vi "MECANISMO BOMBA DE AGUA.vi"() -> ()   [LabVIEW 2021]
uses:
  <vilib>/Instr/_visa.llb/VISA Configure Serial Port (Instr).vi
  <vilib>/MakerHub/LINX/Public/Utilities/Open Serial.vi
  <vilib>/LabVIEW Interface for Arduino/LabVIEW Interface for Arduino.lvlib
  <vilib>/MakerHub/LINX/LMH-LINX.lvlib
  <vilib>/MakerHub/LINX/Public/Sensors/Distance/Ultrasonic/Ultrasonic.lvlib
panel:
  out "HUMEDAD 2":dbl
  in  "VISA resource name":refnum<visa-resource-name>
  out "TEMPERATURA":dbl
  out "HUMEDAD":dbl(knob) scale=0.0..255.0
  out "Centimeters":dbl
  out "Slide":dbl(slide) scale=0.0..500.0
  out "BOMBA (6)":bool
  in  "Boolean 4":bool
  out "VALVULA (8)":bool
  in  "Boolean":bool
  out "VALVULA (7)":bool
  in  "stop":bool
  in  "VISA resource":refnum<visa-resource-name>
  # "VÁLVULA 1"
  # "BOMBA DE AGUA"
  # "VÁLVULA 2"
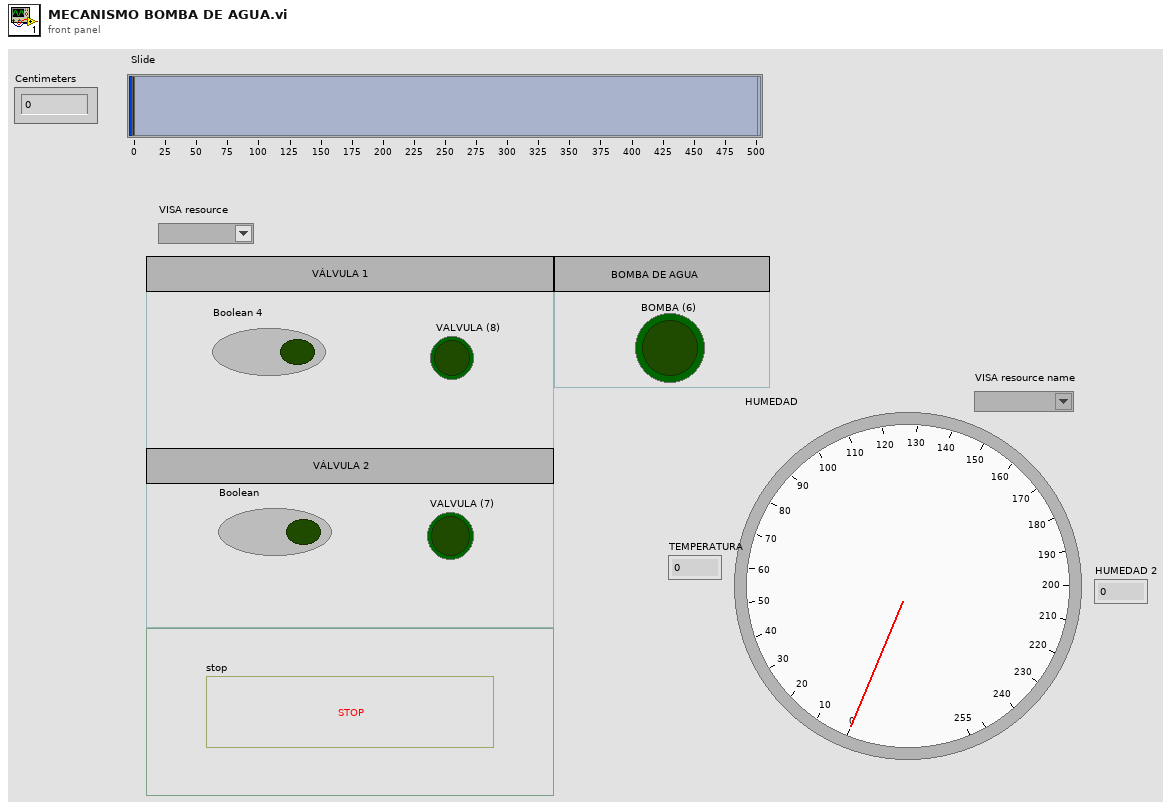
[diagram p1: front panel]
types:
  T1 = typedef "LabVIEW Interface for Arduino.lvlib/Arduino Resource.ctl" = cluster{"VISA resource":refnum<visa-resource-name>, "Board Type":T2, "Connection Type":enum8{"USB / Serial"}, "Bytes Per Packet (15)":u8}
  T2 = typedef "LabVIEW Interface for Arduino.lvlib/Board Type.ctl" = enum16{"Uno", "Dimuelanove w/Atmega 328", "Mega 2560"}
  T3 = typedef "LMH-LINX.lvlib/LINX Ref.ctl" = cluster{"IO":T4, "Interface":T5, "LINX Device Config":T6}
  T4 = typedef "LMH-LINX.lvlib/Platform.ctl" = enum16{"Remote", "Local"}
  T5 = typedef "LMH-LINX.lvlib/Interface.ctl" = enum16{"Serial", "TCP"}
  T6 = typedef "LMH-LINX.lvlib/Device.lvlib/LINX Device Config.ctl" = cluster{"Interface":T5, "COM Port":refnum<visa-resource-name>, "TCP Configuration":T7, "Device Family":u8, "Device ID":u8, "Device Name":string, "TCP Ref":refnum<k5>, "Channels":T8}
  T7 = typedef "LMH-LINX.lvlib/Device.lvlib/TCP Config.ctl" = cluster{"IP Address":string, "Port":u16}
  T8 = typedef "LMH-LINX.lvlib/Channels.ctl" = cluster{"DI":u8[], "DO":u8[], "AI":u8[], "AO":u8[], "PWM":u8[], "QE":u8[], "UART":u8[], "I2C 2":u8[], "SPI":u8[], "CAN":u8[], "Servo":u8[], "AI Ref (V)":dbl, "AI Resolution (Bits)":u8, "AO Ref (V)":dbl, "AO Resolution (Bits)":u8}
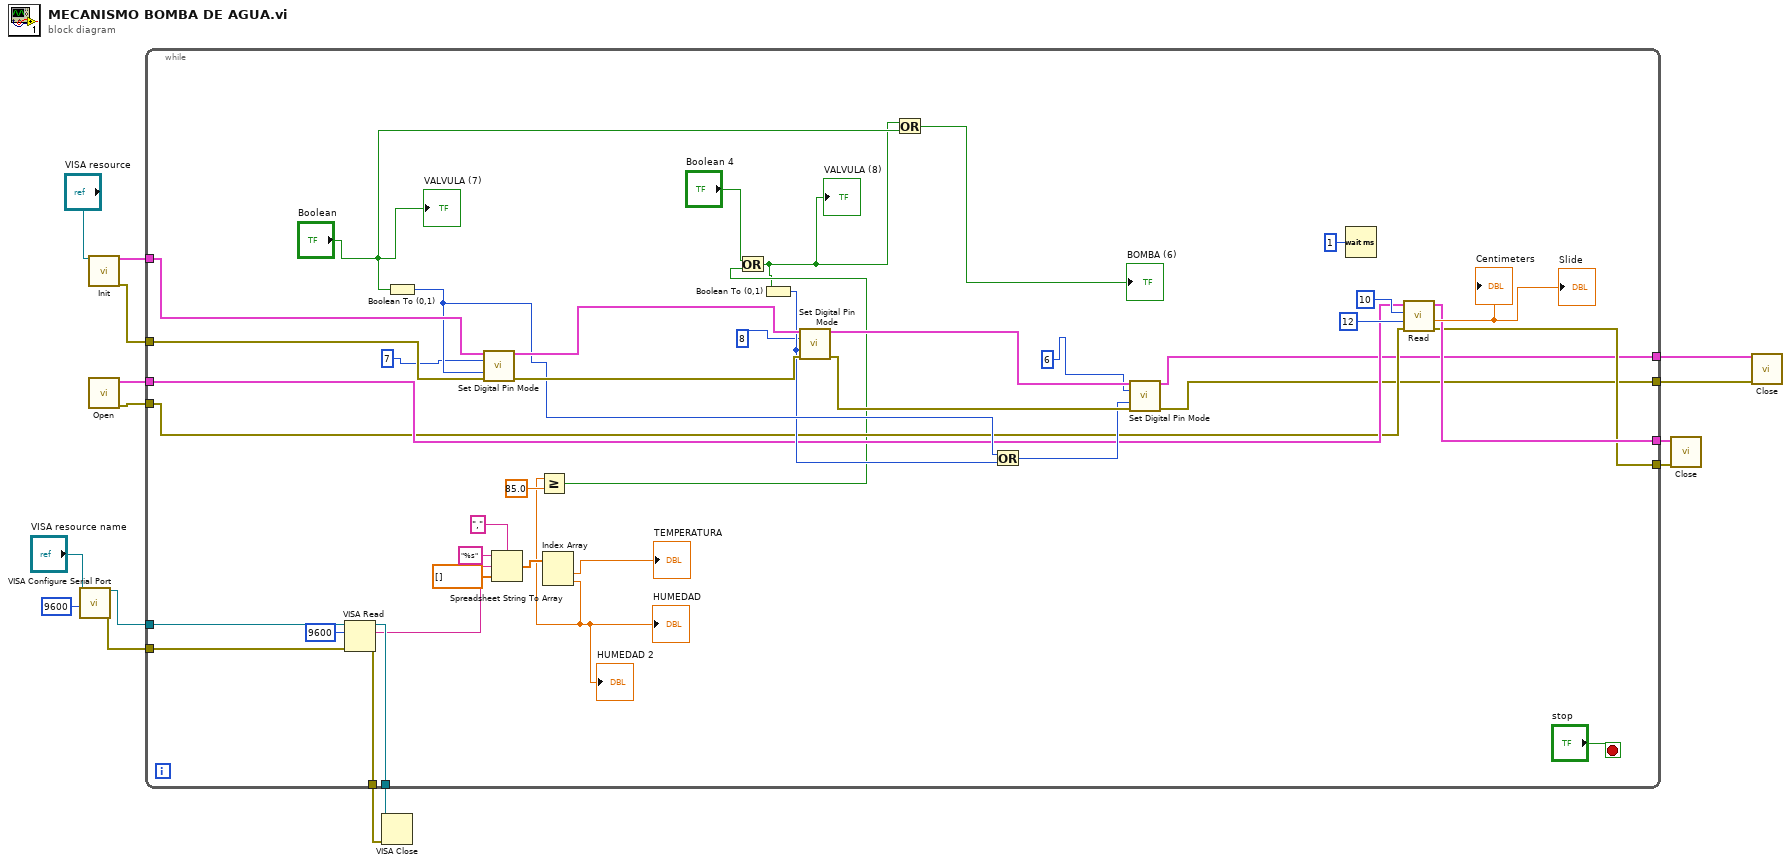
[diagram p0: block diagram]
diagram:
  n1 = call-poly "VISA Configure Serial Port"("VISA resource name"="VISA resource name", "baud rate (9600)"=u32 9600) -> ("VISA resource name out"=w6:refnum<visa-resource-name>, "error out"=w3:errorcluster)  [unwired: 12 in]
  n2 = call <vilib>:"Init.vi"("VISA resource"="VISA resource") -> ("Arduino Resource"=w14:T1, "error out"=w13:errorcluster)  [unwired: 17 in]
  n3 = call-poly <vilib>:"Open.vi"() -> ("Error Out"=w12:errorcluster, "LINX Resource"=w11:T3)  [unwired: 9 in, 1 out]
  n4 = while {
    tunnel: w14 -> [w55]
    tunnel: w13 -> [w54]
    tunnel: w12 -> [w40]
    tunnel: w11 -> [w41]
    tunnel: [w39] -> w10
    tunnel: [w38] -> w9
    tunnel: [w37] -> w8
    tunnel: [w36] -> w7
    tunnel: w6 -> [w35]
    tunnel: [w34] -> w5
    tunnel: [w33] -> w4
    tunnel: w3 -> [w32]
    stop <- "stop" stop-if-true
    n5 = VISA Read(VISA resource name=w35, byte count=u32 9600, error in (no error)=w32) -> (VISA resource name out=w33:refnum<visa-resource-name>, read buffer=w31:string, error out=w34:errorcluster)  [unwired: 1 out]
    n6 = Boolean To (0,1)(Boolean="Boolean") -> (0, 1=w49:i16)
    n7 = call <vilib>:"Set Digital Pin Mode.vi"("Arduino Resource"=w55, "Digital I/O Pin"=u8 7, "Pin Mode (Input)"=w49, "error in"=w54) -> ("Arduino Resource"=w53:T1, "error out"=w52:errorcluster)  [unwired: 10 in]
    n8 = Spreadsheet String To Array(delimiter (Tab)=",", format string="%s", spreadsheet string=w31, array type (2D Dbl)=dbl[] []) -> (array=w27:dbl[])
    n9 = Index Array(array=w27) -> (element #1=→"TEMPERATURA":dbl, element #2=w23:dbl)  [unwired: 2 in]
    "HUMEDAD" <- w23
    "HUMEDAD 2" <- w23
    n10 = Greater Or Equal?(x=w23, y=85.0) -> (x >= y?=w18:bool)
    n11 = Or(x="Boolean 4", y=w18) -> (x .or. y?=w16:bool)
    "VALVULA (8)" <- w16
    n12 = Boolean To (0,1)(Boolean=w16) -> (0, 1=w48:i16)
    n13 = call <vilib>:"Set Digital Pin Mode.vi"("Arduino Resource"=w53, "Digital I/O Pin"=u8 8, "Pin Mode (Input)"=w48, "error in"=w52) -> ("Arduino Resource"=w50:T1, "error out"=w51:errorcluster)  [unwired: 10 in]
    n14 = Or(x=w16, y="Boolean") -> (x .or. y?=→"BOMBA (6)":bool)
    n15 = Or(x=w49, y=w48) -> (x .or. y?=w47:i16)
    n16 = call <vilib>:"Set Digital Pin Mode.vi"("Arduino Resource"=w50, "Digital I/O Pin"=u8 6, "Pin Mode (Input)"=w47, "error in"=w51) -> ("Arduino Resource"=w37:T1, "error out"=w36:errorcluster)  [unwired: 10 in]
    n17 = Wait (ms)(milliseconds to wait=u32 1) -> ()  [unwired: 1 out]
    n18 = call <vilib>:"Read.vi"("Error In"=w40, "DO Channel"=u8 12, "DI Channel"=u8 10, "LINX Resource"=w41) -> ("Error Out"=w38:errorcluster, "Centimeters"=→"Centimeters" →"Slide":dbl, "LINX Resource"=w39:T3)  [unwired: 4 in, 1 out]
    "VALVULA (7)" <- "Boolean"
  }
  n19 = VISA Close(VISA resource name=w4, error in (no error)=w5) -> ()  [unwired: 1 out]
  n20 = call <vilib>:"Close.vi"("Error In"=w9, "LINX Resource"=w10) -> ()  [unwired: 9 in, 1 out]
  n21 = call <vilib>:"Close.vi"("Arduino Resource"=w8, "error in"=w7) -> ()  [unwired: 13 in, 1 out]
